vi "Stem Point Size Write.vi"(4 "error in (no error)":errorcluster, 5 "Value":sgl, 6 "Container State":T3, 7 "Display State In":T1) -> (0 "error out":errorcluster, 3 "Display State Out":T1)   [LabVIEW 2020, in "3D Stem.xctl"]
uses:
  <vilib>/Math Plots/3D Math Plots/3D Stem/3D Stem XCtrl/3D Stem.xctl
  <vilib>/_xctls/Container State.ctl
  <vilib>/Math Plots/3D Math Plots/3D Stem/3D Stem XCtrl/State.ctl
  <vilib>/Math Plots/3D Math Plots/3D Stem/3D Stem/3D Stem.lvclass
  e:/builds/penguin/labview/branches/2020/dev/dist/vi.lib/Math Plots/3D Math Plots/3D Plot/3D Plot/3D Plot.lvclass
  <vilib>/Math Plots/3D Math Plots/3D Plot/Action String/3DMathPlot Ctrl Act Queue.ctl
  <vilib>/Math Plots/3D Math Plots/3D Plot/Action String/3DMathPlot Ctrl Act Cluster.ctl
  <vilib>/Math Plots/3D Math Plots/3D Plot/Action String/3DMathPlot State Class.ctl
  <vilib>/Math Plots/3D Math Plots/3D Plot/3D Plot/3D Plot.lvclass
  <vilib>/_xctls/XControlSupport.lvlib
panel:
  # "Replace the Value Control below with a Control of desired type.\nDo not remove this Control or the others from the connector pane.\nDo not change the connector pane pattern.\nThe Value control should always be the third terminal from top on the input side in the connector pane."
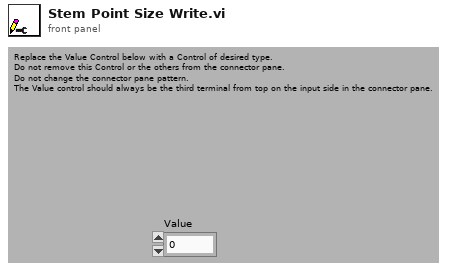
[diagram p1: front panel]
types:
  T1 = typedef "3D Stem.xctl/State.ctl" = cluster{"3D Stem.lvclass":refnum<class "3D Stem.lvclass">, "Control Ref Queue":T2, "Main Frame Color":u32, "Ramp Palette Color":u32, "Projection Palette Color":u32}
  T2 = typedef "3DMathPlot Ctrl Act Queue.ctl" = refnum<queue>
  T3 = typedef "XControlSupport.lvlib/Container State.ctl" = cluster{"Indicator?":bool, "Run Mode?":bool, " Refnum":refnum<vi>}
  T4 = typedef "3DMathPlot State Class.ctl" = enum16{"Update All Objects (Undo)", "Update Light Object Only", "Update Axis Object Only", "Update Plot Object Only", "Update Cursor Object Only", "Update Axis Plot Cursor Objects", "No Update"}
  T5 = typedef "3D Stem.lvclass/3D Stem Property Array.ctl" = T6[]
  T6 = typedef "3D Stem.lvclass/3D Stem Property.ctl" = cluster{"General Property":cluster{"Plot Name":string, "Coordinate System":enum16{"Cartesian", "Cylindrical", "Spherical"}, "Opacity":sgl}, "Projection Property":cluster{"Draw XY":bool, "Draw YZ":bool, "Draw XZ":bool}, "Plot Property":cluster{"Sprite Type":T7, "Point Size":sgl, "Color Ramp Cluster":T8, "Line Style":T9, "Line Width":sgl, "Line Color":u32, "Antialiasing":bool}}
  T7 = typedef "3D Plot.lvclass/Sprite Type.ctl" = enum16{"None", "Empty Square", "Solid Square", "Empty Diamond", "Solid Diamond", "Empty Circle", "Solid Circle", "Asterisk", "Bold X", "Wireframe Sphere", "Solid Sphere", "Wireframe Cube", "Solid Cube"}
  T8 = typedef "3D Plot.lvclass/Color Ramp Cluster.ctl" = cluster{"Color Ramp Style":enum16{"None", "Shaded", "Color spectrum", "Grey scale", "Custom"}, "Color Ramp Array":u32[], "Color Ramp Index":i32[], "Interpolate?":bool, "Logarithm?":bool}
  T9 = typedef "3D Plot.lvclass/Line Type.ctl" = enum16{"None", "Solid", "Dash", "Dot", "Dash Dot"}
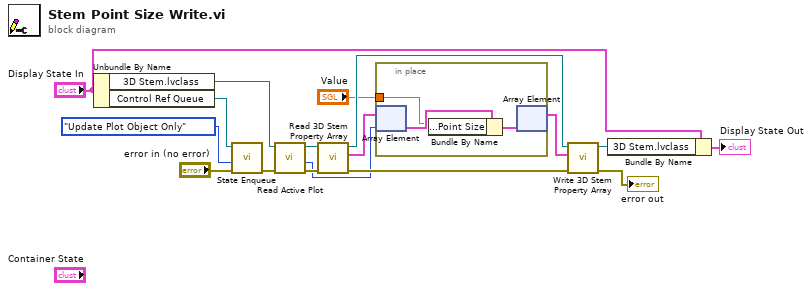
[diagram p0: block diagram]
diagram:
  n1 = Unbundle By Name("Display State In") -> ("3D Stem.lvclass"=w17:refnum<class "3D Stem.lvclass">, "Control Ref Queue"=w4:T2)
  n2 = call <vilib>:"State Enqueue.vi"("error in (no error)"="error in (no error)", "Display State Change Class"=3DMathPlot_State_Class."Update Plot Object Only", "Control Ref Queue"=w4) -> ("error out"=w2:errorcluster)  [unwired: 8 out]
  n3 = call <vilib>:"Read Active Plot.vi"("error in (no error)"=w2, "3D Plot.lvclass in"=w17) -> ("error out"=w15:errorcluster, "Active Plot"=w9:i32, "3D Plot.lvclass out"=w16:refnum<class "3D Stem.lvclass">)  [unwired: 7 out]
  n4 = call <vilib>:"Read 3D Stem Property Array.vi"("error in (no error)"=w15, "3D Stem.lvclass in"=w16) -> ("error out"=w11:errorcluster, "3D Stem Property Array"=w14:T5, "3D Stem.lvclass out"=w13:refnum<class "3D Stem.lvclass">)  [unwired: 7 out]
  n5 = in-place {
    in-place-border: "Value" -> [w18]
    n6 = in-place-array #1(w14, w9) -> (w20:T6)
    n7 = Bundle By Name(cluster=w20, "Plot Property.Point Size"=w18) -> (w19:T6)
    n8 = in-place-array #1(w19) -> (w12:T5)  [unwired: 1 out]
  }
  n9 = call <vilib>:"Write 3D Stem Property Array.vi"("error in (no error)"=w11, "3D Stem Property Array"=w12, "3D Stem.lvclass in"=w13) -> ("error out"=→"error out":errorcluster, "3D Stem.lvclass out"=w10:refnum<class "3D Stem.lvclass">)  [unwired: 7 out]
  n10 = Bundle By Name(cluster="Display State In", "3D Stem.lvclass"=w10) -> (→"Display State Out":T1)
